vi "IsHover Shape.vi"(8 "error in (no error)":errorcluster, 10 "Coords":T1, 11 "Shape in":refnum<data-value>[](array[refnum])) -> (0 "error out":errorcluster, 1 "Node ID":i32, 2 "Found?":bool, 3 "Shape out":refnum<data-value>[](array[refnum]), 4 "Direction":string, 5 "Edge":bool)   [LabVIEW 2017, in "LV Image Editor Framework.lvlib" / "Shape.lvclass"]
uses:
  Shape.lvclass
  <vilib>/Utility/miscctls.llb/LVPoint32TypeDef.ctl
  Read Bounds.vi
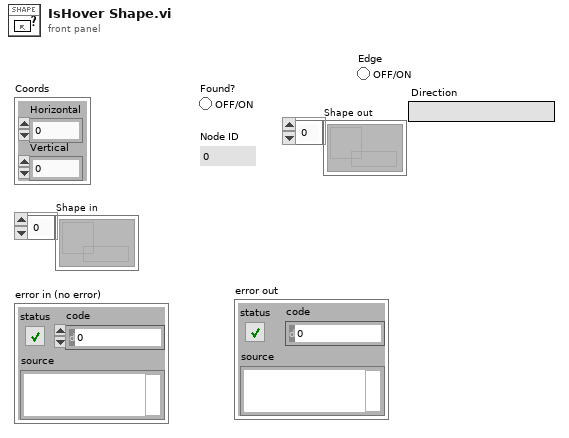
[diagram p1: front panel]
types:
  T1 = typedef "LVPoint32TypeDef.ctl" = cluster{"Horizontal":i32, "Vertical":i32}
  T2 = cluster{"Left":i32, "Top":i32, "Right":i32, "Bottom":i32}
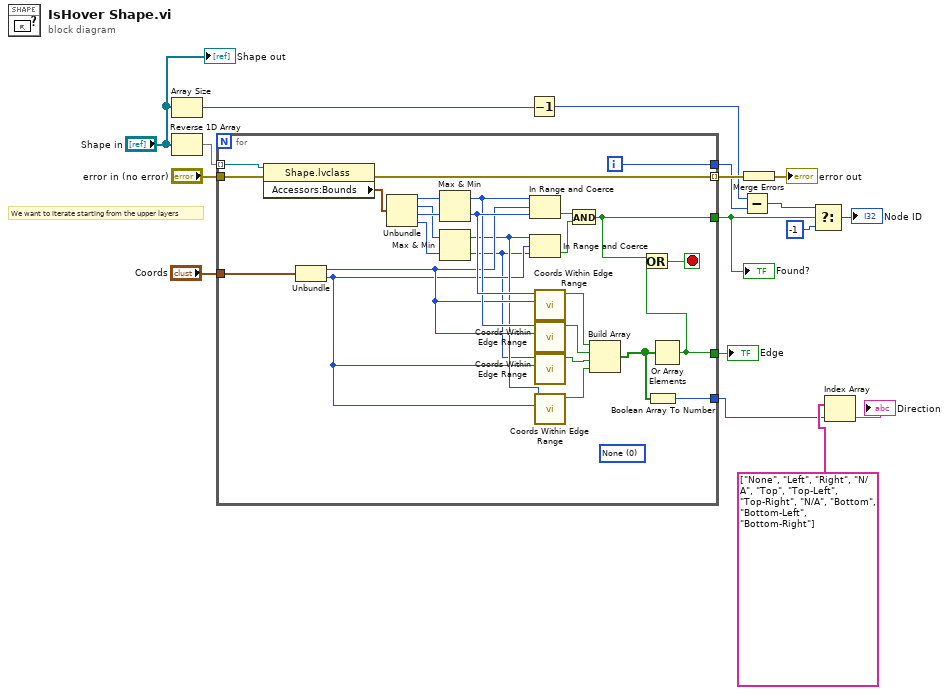
[diagram p0: block diagram]
diagram:
  # "We want to iterate starting from the upper layers"
  n1 = Array Size(array="Shape in") -> (size(s)=w8:i32)
  n2 = Reverse 1D Array(array="Shape in") -> (reversed array=w10:refnum<data-value>[])
  n3 = for {
    tunnel: "Coords" -> [w38]
    tunnel: [w22] -> w13
    tunnel: [w44] -> w6
    tunnel: w10 -> [w43] mode=indexing
    tunnel: [w42] -> w15 mode=indexing
    tunnel: "error in (no error)" -> [w41]
    tunnel: [w21] -> w4
    tunnel: [w18] -> w2
    i -> [w44]
    stop <- w20 stop-if-true
    (unwired) u16 0 items=["None"=0, "Left"=1, "Right"=2, "Top"=4, "Top-Left"=5, "Top-Right"=6, "Bottom"=8, "Bottom-Left"=9, "Bottom-Right"=10]
    n4 = property class="Shape.lvclass"(reference=w43, error in=w41) -> (error out=w42:errorcluster, "Accessors:Bounds"=w33:T2)  [unwired: 1 out]
    n5 = Unbundle(w38) -> ("Horizontal"=w30:i32, "Vertical"=w28:i32)
    n6 = Unbundle(w33) -> ("Left"=w40:i32, "Top"=w37:i32, "Right"=w39:i32, "Bottom"=w36:i32)
    n7 = Max & Min(x=w40, y=w39) -> (max(x,y)=w31:i32, min(x,y)=w32:i32)
    n8 = Max & Min(x=w37, y=w36) -> (max(x,y)=w29:i32, min(x,y)=w27:i32)
    n9 = In Range and Coerce(upper limit=w31, x=w30, lower limit=w32) -> (In Range?=w35:bool)  [unwired: 1 out]
    n10 = In Range and Coerce(upper limit=w29, x=w28, lower limit=w27) -> (In Range?=w34:bool)  [unwired: 1 out]
    n11 = call "Coords Within Edge Range.vi"("Horizontal"=w30, "Numeric"=w32) -> ("Boolean"=w26:bool)  [unwired: 9 in]
    n12 = call "Coords Within Edge Range.vi"("Horizontal"=w30, "Numeric"=w31) -> ("Boolean"=w25:bool)  [unwired: 9 in]
    n13 = call "Coords Within Edge Range.vi"("Horizontal"=w28, "Numeric"=w27) -> ("Boolean"=w24:bool)  [unwired: 9 in]
    n14 = call "Coords Within Edge Range.vi"("Horizontal"=w28, "Numeric"=w29) -> ("Boolean"=w23:bool)  [unwired: 9 in]
    n15 = And(x=w35, y=w34) -> (x .and. y?=w22:bool)
    n16 = Build Array(w26, w25, w24, w23) -> (w19:bool[])
    n17 = Boolean Array To Number(Boolean array=w19) -> (number=w18:u32)
    n18 = Or Array Elements(Boolean array=w19) -> (logical OR=w21:bool)
    n19 = Or(x=w22, y=w21) -> (x .or. y?=w20:bool)
  }
  "Found?" <- w13
  "Edge" <- w4
  n20 = Decrement(x=w8) -> (x-1=w7:i32)
  n21 = Subtract(x=w7, y=w6) -> (x-y=w5:i32)
  n22 = Merge Errors(w15) -> (→"error out":errorcluster)
  n23 = Select(t=w5, s=w13, f=-1) -> (s? t:f=→"Node ID":i32)
  n24 = Index Array(array=string[] ["None", "Left", "Right", "N/A", "Top", "Top-Left", "Top-Right", "N/A", "Bottom", "Bottom-Left", "Bottom-Right"], index=w2) -> (element=→"Direction":string)
  "Shape out" <- "Shape in"
